vi "SCAN.vi"(4 "count":i64, 6 "MATCH pattern":string, 7 "TYPE":string, 8 "error in (no error)":errorcluster, 9 "cursor":i64, 11 "Redis Client in":refnum<class "Redis Client.lvclass">) -> (0 "error out":errorcluster, 2 "RESP3 Value":variant, 3 "Redis Client out":refnum<class "Redis Client.lvclass">)   [LabVIEW 2019, in "Redis Client for LabVIEW.lvlib" / "Redis Client.lvclass"]
uses:
  Redis Client.lvclass
  lib/RESP3-for-LabVIEW/RESP3/subVIs/RESP3 Make String Base.vi
  lib/RESP3-for-LabVIEW/RESP3/types/RESP3 data type attribute.vi
  lib/RESP3-for-LabVIEW/RESP3/RESP3.lvlib
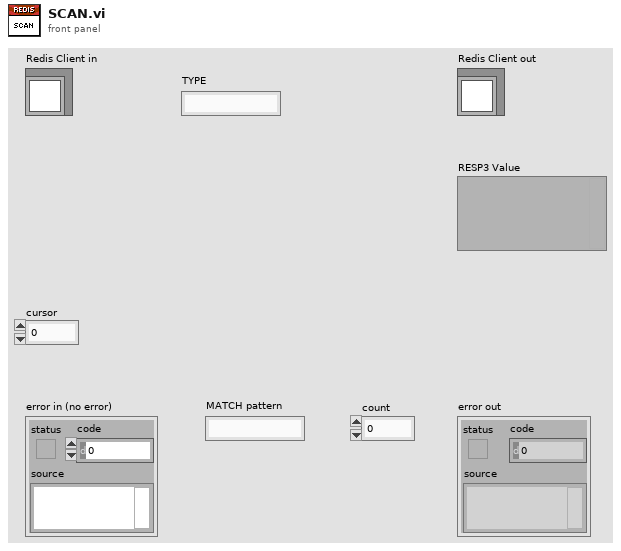
[diagram p1: front panel]
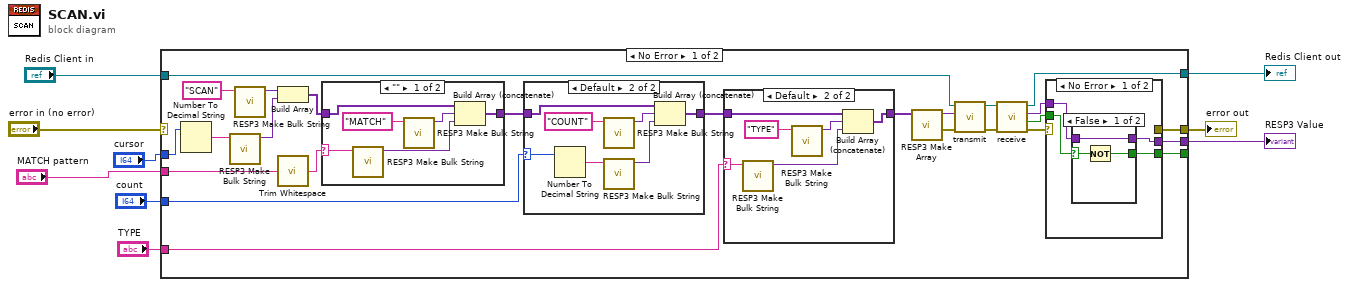
[diagram p0: block diagram]
diagram:
  n1 = case shown="No Error" "error in (no error)" {
    selector: "error in (no error)" -> [_ w66]
    tunnel: [w23 w66] -> w8
    tunnel: "Redis Client in" -> [w34 w65]
    tunnel: [w32 w65] -> w6
    tunnel: "cursor" -> [w29 _]
    tunnel: [w22 _] -> _
    tunnel: [w19 _] -> w4
    tunnel: "MATCH pattern" -> [w17 _]
    tunnel: "count" -> [w14 _]
    tunnel: "TYPE" -> [w12 _]
    frame No Error {
      n2 = Number To Decimal String(number=w29) -> (decimal integer string=w18:string)  [unwired: 1 in]
      n3 = call "RESP3 Make Bulk String.vi"("String"=w18) -> ("RESP3 Value out"=w27:variant)  [unwired: 9 in, 1 out]
      n4 = call "RESP3 Make Bulk String.vi"("String"="SCAN" ("string in")) -> ("RESP3 Value out"=w28:variant)  [unwired: 9 in, 1 out]
      n5 = Build Array(w28, w27) -> (w15:variant[])
      n6 = call <vilib>:"Trim Whitespace.vi"("string"=w17) -> ("trimmed string"=w16:string)  [unwired: 1 in]
      n7 = case shown="\"\"" w16 {
        selector: w16 -> [w54 _]
        tunnel: w15 -> [w53 w56]
        tunnel: [w50 w56] -> w13
        frame "" {
          n8 = call "RESP3 Make Bulk String.vi"("String"=w54) -> ("RESP3 Value out"=w51:variant)  [unwired: 9 in, 1 out]
          n9 = call "RESP3 Make Bulk String.vi"("String"="MATCH") -> ("RESP3 Value out"=w52:variant)  [unwired: 9 in, 1 out]
          n10 = Build Array (concatenate)(w53, w52, w51) -> (w50:variant[])
        }
        frame Default {
        }
      }
      n11 = case shown="Default" w14 {
        selector: w14 -> [_ w48]
        tunnel: [w42 w45] -> w11
        tunnel: w13 -> [w42 w47]
        frame ..0 {
        }
        frame Default {
          n12 = Number To Decimal String(number=w48) -> (decimal integer string=w49:string)  [unwired: 1 in]
          n13 = call "RESP3 Make Bulk String.vi"("String"="COUNT") -> ("RESP3 Value out"=w44:variant)  [unwired: 9 in, 1 out]
          n14 = call "RESP3 Make Bulk String.vi"("String"=w49) -> ("RESP3 Value out"=w46:variant)  [unwired: 9 in, 1 out]
          n15 = Build Array (concatenate)(w47, w44, w46) -> (w45:variant[])
        }
      }
      n16 = case shown="Default" w12 {
        selector: w12 -> [_ w36]
        tunnel: [w35 w39] -> w10
        tunnel: w11 -> [w35 w41]
        frame "" {
        }
        frame Default {
          n17 = call "RESP3 Make Bulk String.vi"("String"=w36) -> ("RESP3 Value out"=w40:variant)  [unwired: 9 in, 1 out]
          n18 = call "RESP3 Make Bulk String.vi"("String"="TYPE") -> ("RESP3 Value out"=w38:variant)  [unwired: 9 in, 1 out]
          n19 = Build Array (concatenate)(w41, w38, w40) -> (w39:variant[])
        }
      }
      n20 = call "RESP3 Make Array.vi"("RESP3 Values in"=w10) -> ("error out"=w25:errorcluster, "RESP3 Value out"=w26:variant)  [unwired: 9 in]
      n21 = call-dynamic "transmit.vi"("error in (no error)"=w25, "RESP3 Value"=w26, "Redis Client in"=w34) -> ("error out"=w31:errorcluster, "Redis Client out"=w33:refnum<class "Redis Client.lvclass">)  [unwired: 7 in]
      n22 = call-dynamic "receive.vi"("error in (no error)"=w31, "Redis Client in"=w33) -> ("error out"=w21:errorcluster, "timed out?"=w20:bool, "RESP3 Value"=w24:variant, "Redis Client out"=w32:refnum<class "Redis Client.lvclass">)  [unwired: 6 in]
      n23 = case shown="No Error" w21 {
        selector: w21 -> [_ w64]
        tunnel: w24 -> [w60 _]
        tunnel: [_ w64] -> w23
        tunnel: [w59 _] -> w22
        tunnel: w20 -> [w58 _]
        tunnel: [w57 _] -> w19
        frame No Error {
          n24 = case shown="False" w58 {
            selector: w58 -> [w61 _]
            tunnel: w60 -> [w62 _]
            tunnel: [w63 _] -> w59
            tunnel: [w62 _] -> w57
            frame False {
              n25 = Not(x=w61) -> (.not. x?=w63:bool)
            }
            frame True {
            }
          }
        }
        frame Error {
        }
      }
    }
    frame Error {
    }
  }
  "error out" <- w8
  "Redis Client out" <- w6
  "RESP3 Value" <- w4
